vi "get_data_folder_path.vi"(8 "error in (no error)":errorcluster, 11 "GenericComponent in":refnum<class "GenericComponent.lvclass">) -> (0 "error out":errorcluster, 2 "data folder path":path, 3 "GenericComponent out":refnum<class "GenericComponent.lvclass">)   [LabVIEW 2010, in "GenericComponent.lvclass"]
uses:
  GenericComponent.lvclass
  class_data.vi
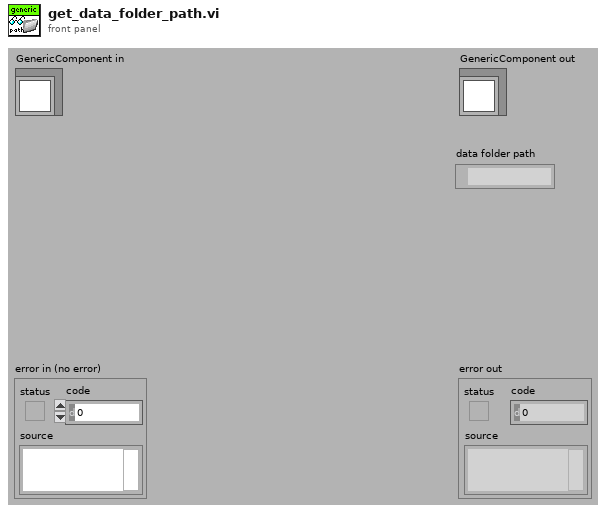
[diagram p1: front panel]
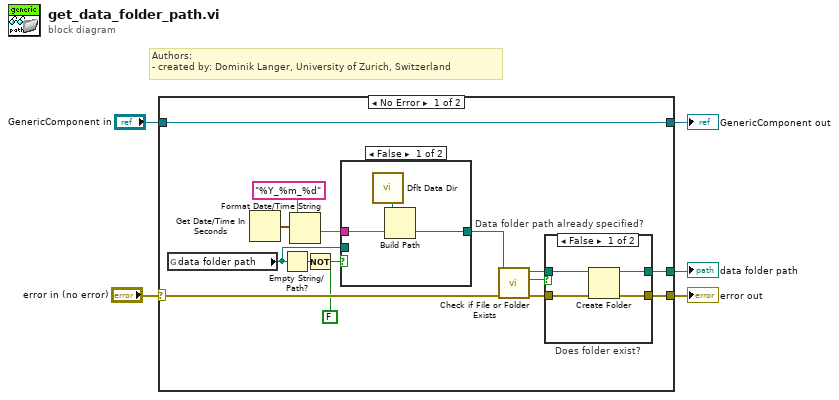
[diagram p0: block diagram]
diagram:
  # "Authors: \n- created by: Dominik Langer, University of Zurich, Switzerland"
  n1 = case shown="No Error" "error in (no error)" {
    selector: "error in (no error)" -> [w10 w31]
    tunnel: [w7 w31] -> w4
    tunnel: [w19 w30] -> w2
    tunnel: "GenericComponent in" -> [w19 w30]
    tunnel: [w8 _] -> w1
    frame No Error {
      n2 = global read "class_data.vi" "data folder path"() -> (w15:path)
      n3 = Get Date/Time In Seconds() -> (seconds since 1Jan1904=w16:timestamp)
      n4 = Empty String/Path?(string/path=w15) -> (empty?=w17:bool)
      n5 = Format Date/Time String(time format string (%c)="%Y_%m_%d", seconds (now)=w16) -> (date/time string=w18:string)  [unwired: 1 out]
      n6 = Not(x=w17) -> ()  [unwired: 1 out]
      n7 = case "Data folder path already specified?" shown="False" FALSE {
        tunnel: w18 -> [w27 _]
        tunnel: [w26 w29] -> w9
        tunnel: w15 -> [_ w29]
        frame False {
          n8 = call <vilib>:"Dflt Data Dir.vi"() -> ("App:Default Data Directory"=w28:path)
          n9 = Build Path(base path=w28, name or relative path=w27) -> (appended path=w26:path)
        }
        frame True {
        }
      }
      n10 = call <vilib>:"Check if File or Folder Exists.vi"("error in (no error)"=w10, "path"=w9) -> ("error out"=w11:errorcluster, "file or folder exists?"=w12:bool, "dup path"=w13:path)  [unwired: 7 out]
      n11 = case "Does folder exist?" shown="False" w12 {
        tunnel: w11 -> [w23 w25]
        tunnel: w13 -> [w21 w24]
        tunnel: [w22 w25] -> w7
        tunnel: [w20 w24] -> w8
        frame False {
          n12 = Create Folder(path (use dialog)=w21, error in=w23) -> (created path=w20:path, error out=w22:errorcluster)  [unwired: 2 out]
        }
        frame True {
        }
      }
    }
    frame Error {
    }
  }
  "error out" <- w4
  "GenericComponent out" <- w2
  "data folder path" <- w1
